vi "EnFlo_Seeder_Control.vi"(0 "Current Time (s)":dbl) -> ()   [LabVIEW 2016]
panel:
  in  "Minium Seeder power setting (Pmin)":dbl=27.0
  in  "Minimum Transducer Setting (Tmin)":dbl=6.0
  in  "Fluid Flowrate Factor":dbl=1.2 min=0.2 max=4.0 step=0.1 format="%.1g"
  in  "Sugar Strength":dbl=0.23
  out "Leak Detected or Emergency Stop":bool
  in  "Performing hand clean":bool
  out "Run Transducer":bool
  out "Sugar Pump":bool
  out "Low Flow":bool
  out "High Flow":bool
  out "Time Since Last Flush (min)":dbl
  out "Running Flush time":dbl
  out "Transducer setting":dbl
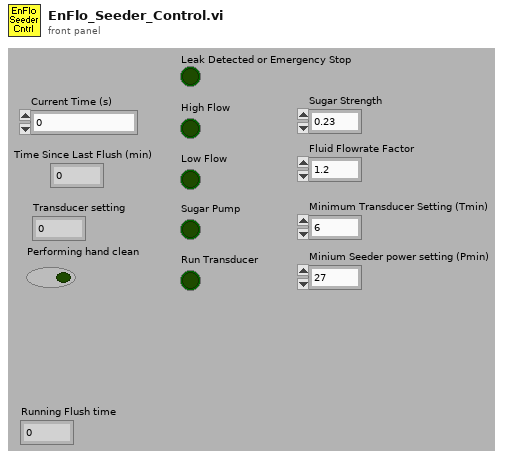
[diagram p1: front panel]
types:
  T1 = typedef "LVDateTimeRec.ctl" = cluster{"fractional second":dbl, "second":i32, "minute":i32, "hour":i32, "day of month":i32, "month":i32, "year":i32, "day of week":i32, "day of year":i32, "DST":i32}
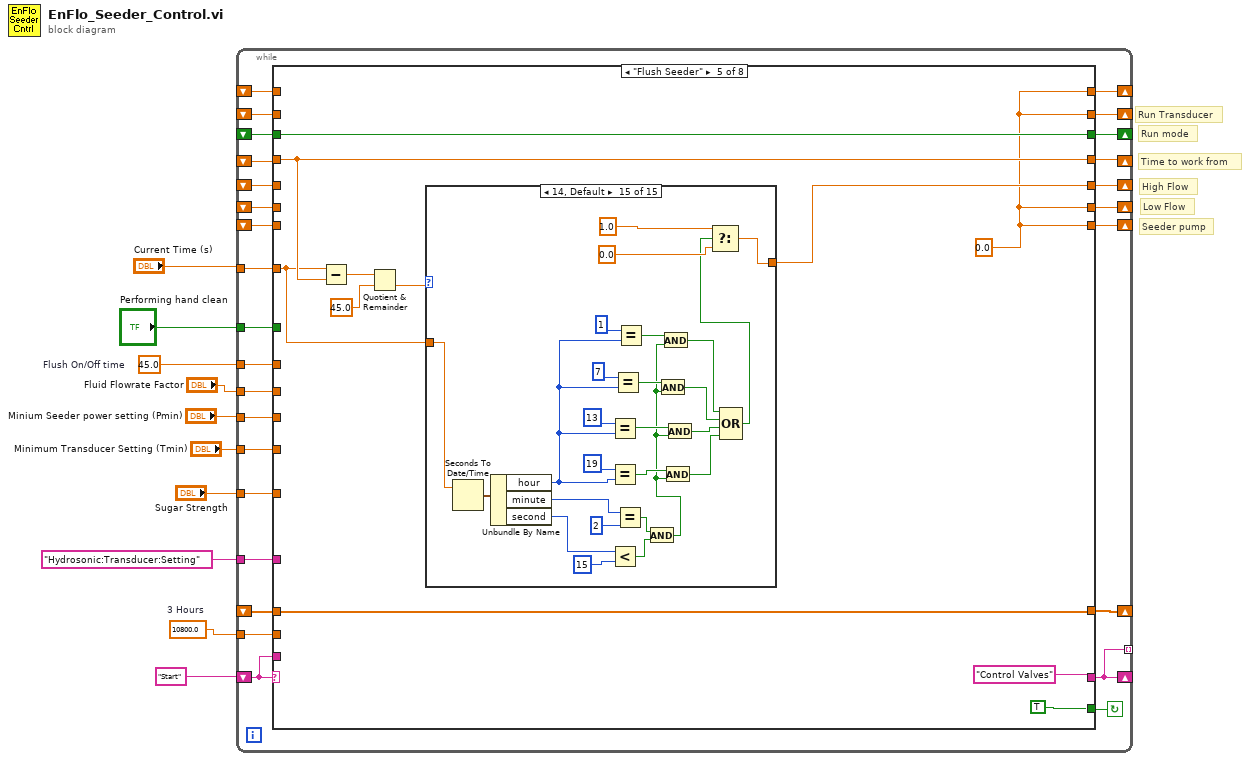
[diagram p0: block diagram]
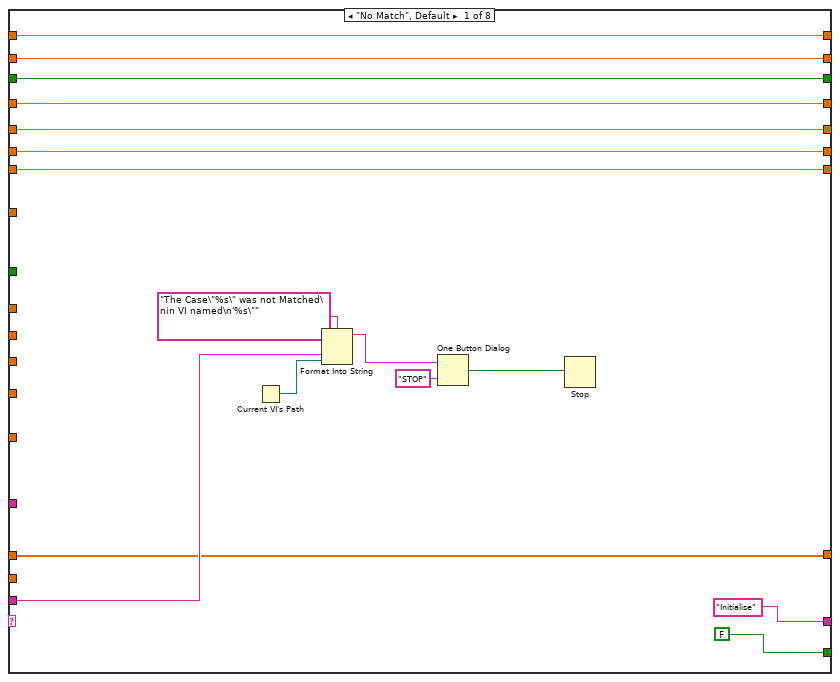
[diagram p2: hidden frame]
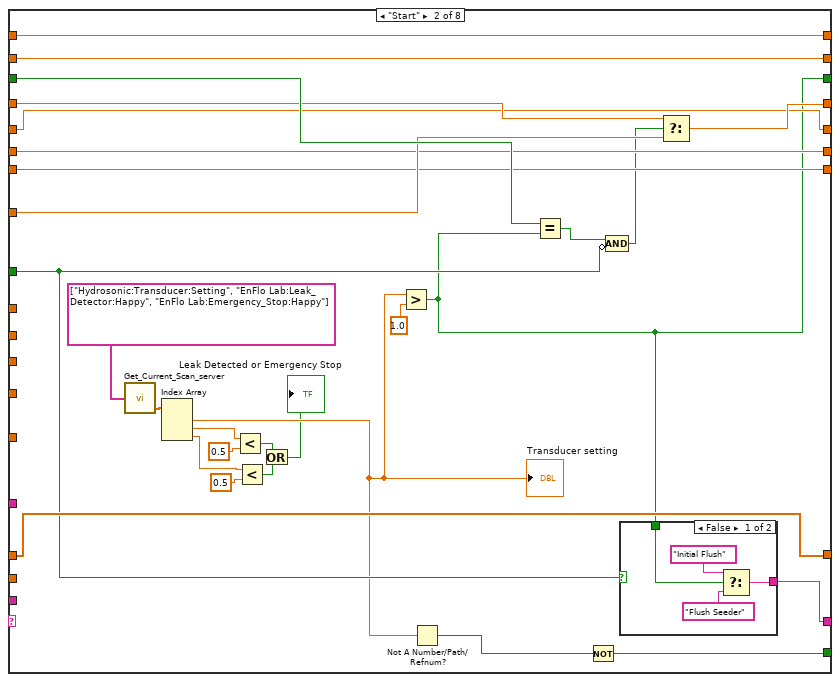
[diagram p3: hidden frame]
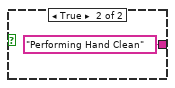
[diagram p4: hidden frame]
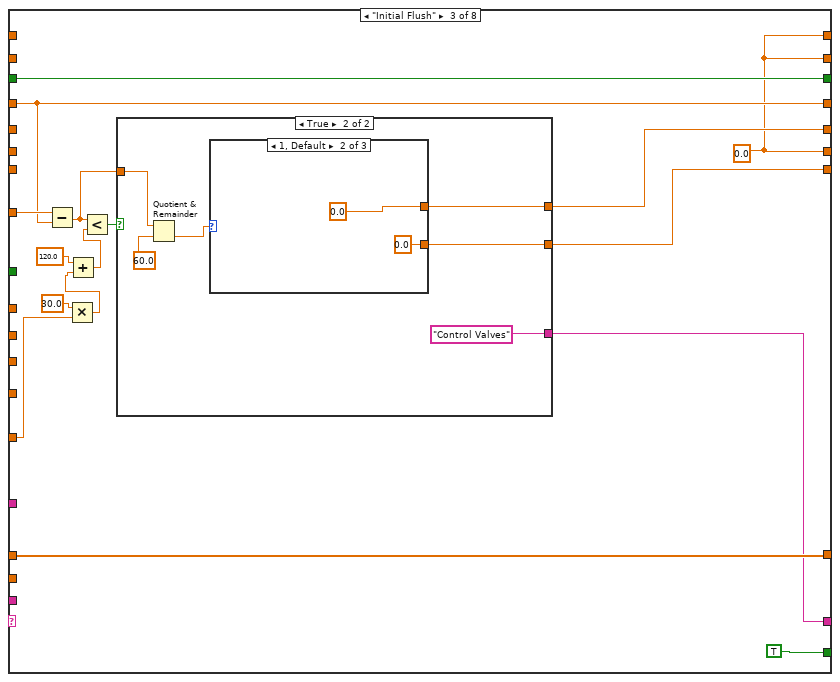
[diagram p5: hidden frame]
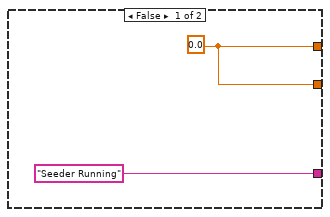
[diagram p6: hidden frame]
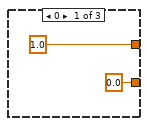
[diagram p7: hidden frame]
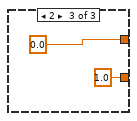
[diagram p8: hidden frame]
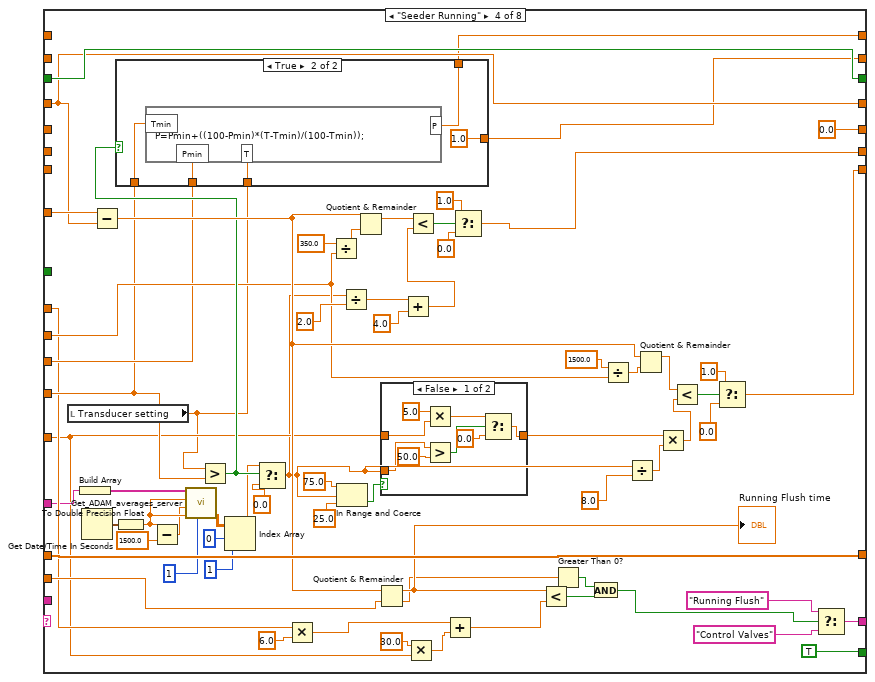
[diagram p9: hidden frame]
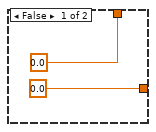
[diagram p11: hidden frame]
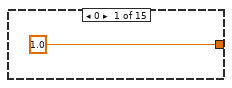
[diagram p12: hidden frame]
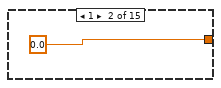
[diagram p13: hidden frame]
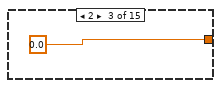
[diagram p14: hidden frame]
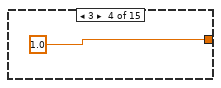
[diagram p15: hidden frame]
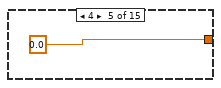
[diagram p16: hidden frame]
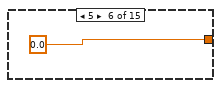
[diagram p17: hidden frame]
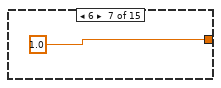
[diagram p18: hidden frame]
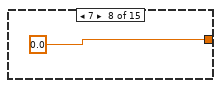
[diagram p19: hidden frame]
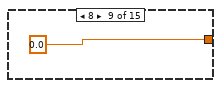
[diagram p20: hidden frame]
diagram:
  w2 = 45.0  # Flush On/Off time
  w8 = 10800.0  # 3 Hours
  # "Run Transducer"
  # "Seeder pump"
  # "Low Flow"
  # "High Flow"
  # "Run mode"
  # "Time to work from"
  n1 = while {
    shift-left: "Start" -> [w37]
    shift-right: [w21] -> _
    shift-right: [w36] -> _
    shift-left: _ -> [w33]
    shift-right: [w35] -> _
    shift-left: _ -> [w34]
    tunnel: "Current Time (s)" -> [w32]
    shift-right: [w30] -> _
    shift-left: _ -> [w31]
    shift-right: [w29] -> _
    shift-left: _ -> [w28]
    shift-right: [w26] -> _
    shift-left: _ -> [w27]
    shift-right: [w24] -> _
    shift-left: _ -> [w25]
    shift-right: [w23] -> _
    shift-left: _ -> [w22]
    tunnel: [w21] -> _ mode=indexing
    tunnel: w8 -> [w20]
    tunnel: "Performing hand clean" -> [w19]
    tunnel: "Sugar Strength" -> [w18]
    shift-right: [w17] -> _
    shift-left: _ -> [w16]
    tunnel: "Fluid Flowrate Factor" -> [w15]
    tunnel: "Minimum Transducer Setting (Tmin)" -> [w14]
    tunnel: "Minium Seeder power setting (Pmin)" -> [w13]
    tunnel: w2 -> [w12]
    tunnel: "Hydrosonic:Transducer:Setting" -> [w11]
    stop <- w38 continue-if-true
    n2 = case shown="\"Flush Seeder\"" w37 {
      tunnel: [FALSE w80 TRUE TRUE TRUE TRUE TRUE FALSE] -> w38
      tunnel: ["Initialise" w75 w94 w164 "Control Valves" "Control Valves" "Control Valves" "End"] -> w21
      tunnel: w37 -> [w49 _ _ _ _ _ _ _]
      tunnel: [w44 w78 w97 w183 w209 w255 w269 w322] -> w36
      tunnel: [w46 w60 w102 w185 w210 w256 w270 w331] -> w35
      tunnel: w34 -> [w46 w79 w102 w185 w210 w256 w270 w331]
      tunnel: w33 -> [w44 w77 w97 w183 w209 w255 w269 w322]
      tunnel: w32 -> [_ w76 w98 w184 w202 _ _ w323]
      tunnel: w31 -> [w45 w74 _ _ _ _ _ w319]
      tunnel: [w45 w74 w101 0.0 w205 w253 w268 w319] -> w30
      tunnel: w28 -> [w43 w72 _ _ _ _ _ w317]
      tunnel: [w43 w72 w88 w173 w203 w253 w264 w317] -> w29
      tunnel: w27 -> [w42 w71 _ _ _ _ _ w315]
      tunnel: [w42 w71 w99 w167 w203 w253 w265 w315] -> w26
      tunnel: w25 -> [w41 w73 w100 w182 w204 w254 w267 w311]
      tunnel: [w41 w73 w100 w182 w204 w254 w267 w304] -> w24
      tunnel: w22 -> [w40 w70 _ _ _ _ _ w313]
      tunnel: [w40 w70 w88 w148 w203 w253 w264 w313] -> w23
      tunnel: w20 -> [_ _ _ w156 _ _ _ w307]
      tunnel: w19 -> [_ w67 _ _ _ _ _ _]
      tunnel: w18 -> [_ _ w91 w123 _ _ _ _]
      tunnel: [w39 w63 w88 w147 w203 w253 w264 w299] -> w17
      tunnel: w16 -> [w39 w63 _ _ _ _ _ w299]
      tunnel: w15 -> [_ _ _ w142 _ _ _ _]
      tunnel: w14 -> [_ _ _ w139 _ _ _ _]
      tunnel: w13 -> [_ _ _ w140 _ _ _ _]
      tunnel: w12 -> [_ _ _ w138 _ _ w263 _]
      tunnel: w11 -> [_ _ _ w135 _ _ _ _]
      frame "No Match", Default {
        n3 = Current VI's Path() -> (path=w48:path)
        n4 = Format Into String(format string="The Case\"%s\" was not Matched\nin VI named\n'%s\"" ("Format String"), w49, w48) -> (resulting string=w52:string)  [unwired: 2 in, 1 out]
        n5 = One Button Dialog(message=w52, button name ("OK")="STOP") -> (true=w50:bool)
        n6 = Stop(stop? (T)=w50) -> ()
      }
      frame "Start" {
        n7 = call "Get_Current_Scan_server.vi"("Desired Channels"=string[] ["Hydrosonic:Transducer:Setting", "EnFlo Lab:Leak_Detector:Happy", "EnFlo Lab:Emergency_Stop:Happy"] ("appended array")) -> ("Numerical Values"=w82:dbl[])  [unwired: 2 out]
        n8 = Index Array(array=w82) -> (element #1=w62:dbl, element #2=w65:dbl, element #3=w58:dbl)  [unwired: 3 in]
        "Transducer setting" <- w62
        n9 = Less?(x=w65, y=0.5) -> (x < y?=w56:bool)
        n10 = Less?(x=w58, y=0.5) -> (x < y?=w57:bool)
        n11 = Or(x=w56, y=w57) -> (x .or. y?=→"Leak Detected or Emergency Stop":bool)
        n12 = Greater?(x=w62, y=1.0) -> (0:w60:bool)
        n13 = Not A Number/Path/Refnum?(number/path/refnum=w62) -> (NaN/Path/Refnum?=w81:bool)
        n14 = Equal?(x=w79, y=w60) -> (x = y?=w69:bool)
        n15 = Not(x=w81) -> (.not. x?=w80:bool)
        n16 = Compound Arithmetic op=AND(w69, invert w67) -> (w68:bool)
        n17 = case shown="False" w67 {
          tunnel: w60 -> [w86 _]
          tunnel: [w85 "Performing Hand Clean"] -> w75
          frame False {
            n18 = Select(t="Initial Flush", s=w86, f="Flush Seeder") -> (s? t:f=w85:string)
          }
          frame True {
          }
        }
        n19 = Select(t=w77, s=w68, f=w76) -> (s? t:f=w78:dbl)
      }
      frame "Initial Flush" {
        w88 = 0.0
        n20 = Subtract(x=w98, y=w97) -> (x-y=w95:dbl)
        n21 = Multiply(x=30.0 ("y"), y=w91) -> (x*y=w90:dbl)
        n22 = Add(x=120.0 ("y"), y=w90) -> (x+y=w89:dbl)
        n23 = Less?(x=w95, y=w89) -> (x < y?=w96:bool)
        n24 = case shown="True" w96 {
          tunnel: [w105 w111] -> w101
          tunnel: [w105 w110] -> w99
          tunnel: w95 -> [_ w108]
          tunnel: ["Seeder Running" "Control Valves"] -> w94
          frame False {
            w105 = 0.0
          }
          frame True {
            n25 = Quotient & Remainder(x=w108, y=60.0) -> (floor(x/y)=w107:dbl)  [unwired: 1 out]
            n26 = case shown="1, Default" w107 {
              tunnel: [1.0 0.0 0.0] -> w111
              tunnel: [0.0 0.0 1.0] -> w110
              frame 0 {
              }
              frame 1, Default {
              }
              frame 2 {
              }
            }
          }
        }
      }
      frame "Seeder Running" {
        n27 = local read "Transducer setting"() -> (w118:dbl)
        n28 = Build Array(w135) -> (w134:string[])
        n29 = Get Date/Time In Seconds() -> (seconds since 1Jan1904=w133:timestamp)
        n30 = Subtract(x=w184, y=w183) -> (x-y=w162:dbl)
        n31 = To Double Precision Float(number=w133) -> (double precision float=w132:dbl)
        n32 = Subtract(x=w132, y=1500.0) -> (x-y=w119:dbl)
        n33 = call "Get_ADAM_averages_server.vi"("No of averages"=1, "End time"=w132, "Start time"=w119, "Clients time"=w132, "ADAM Ch Names"=w134) -> ("DBL values"=w130:dbl[][])  [unwired: 1 in, 4 out]
        n34 = Greater?(x=w118, y=w139) -> (0:w149:bool)
        n35 = case shown="True" w149 {
          tunnel: [0.0 1.0] -> w148
          tunnel: [0.0 w198] -> w147
          tunnel: w140 -> [_ w200]
          tunnel: w139 -> [_ w199]
          tunnel: w118 -> [_ w197]
          frame False {
          }
          frame True {
            n36 = formula code="P=Pmin+((100-Pmin)*(T-Tmin)/(100-Tmin));"("Tmin"=w199, "T"=w197, "Pmin"=w200) -> ("P"=w198:dbl)
          }
        }
        n37 = Index Array(array=w130, index (row)=0, index (col)=1 ("disabled index (col)")) -> (element=w127:dbl)
        n38 = Select(t=w127, s=w149, f=0.0) -> (s? t:f=w121:dbl)
        n39 = Multiply(x=w138, y=6.0) -> (x*y=w136:dbl)
        n40 = Divide(x=350.0 ("y"), y=w142) -> (x/y=w144:dbl)
        n41 = In Range and Coerce(upper limit=75.0, x=w121, lower limit=25.0) -> (In Range?=w124:bool)  [unwired: 1 out]
        n42 = Divide(x=w121, y=2.0) -> (x/y=w146:dbl)
        n43 = Quotient & Remainder(x=w162, y=w144) -> (x-y*floor(x/y)=w181:dbl)  [unwired: 1 out]
        n44 = Quotient & Remainder(x=w162, y=w156) -> (x-y*floor(x/y)=w163:dbl, floor(x/y)=w160:dbl)
        "Running Flush time" <- w163
        n45 = case shown="False" w124 {
          tunnel: w123 -> [w187 w194]
          tunnel: [w191 w194] -> w122
          tunnel: w121 -> [w193 _]
          frame False {
            n46 = Multiply(x=5.0, y=w187) -> (x*y=w188:dbl)
            n47 = Greater?(x=w193, y=50.0) -> (0:w190:bool)
            n48 = Select(t=w188, s=w190, f=0.0) -> (s? t:f=w191:dbl)
          }
          frame True {
          }
        }
        n49 = Add(x=w146, y=4.0) -> (x+y=w176:dbl)
        n50 = Multiply(x=30.0 ("y"), y=w123) -> (x*y=w152:dbl)
        n51 = Less?(x=w181, y=w176) -> (x < y?=w180:bool)
        n52 = Add(x=w136, y=w152) -> (x+y=w151:dbl)
        n53 = Select(t=1.0, s=w180, f=0.0) -> (s? t:f=w173:dbl)
        n54 = Less?(x=w163, y=w151) -> (x < y?=w158:bool)
        n55 = Greater Than 0?(x=w160) -> (x > 0?=w159:bool)
        n56 = And(x=w159, y=w158) -> (x .and. y?=w157:bool)
        n57 = Divide(x=1500.0 ("y"), y=w142) -> (x/y=w141:dbl)
        n58 = Divide(x=w121, y=8.0) -> (x/y=w154:dbl)
        n59 = Quotient & Remainder(x=w162, y=w141) -> (x-y*floor(x/y)=w168:dbl)  [unwired: 1 out]
        n60 = Multiply(x=w122, y=w154) -> (x*y=w155:dbl)
        n61 = Less?(x=w168, y=w155) -> (x < y?=w169:bool)
        n62 = Select(t=1.0, s=w169, f=0.0) -> (s? t:f=w167:dbl)
        n63 = Select(t="Running Flush", s=w157, f="Control Valves") -> (s? t:f=w164:string)
      }
      frame "Flush Seeder" {
        w203 = 0.0
        n64 = Subtract(x=w202, y=w209) -> (x-y=w208:dbl)
        n65 = Quotient & Remainder(x=w208, y=45.0) -> (floor(x/y)=w206:dbl)  [unwired: 1 out]
        n66 = case shown="14, Default" w206 {
          tunnel: [1.0 0.0 0.0 1.0 0.0 0.0 1.0 0.0 0.0 1.0 0.0 0.0 1.0 0.0 w249] -> w205
          tunnel: w202 -> [_ _ _ _ _ _ _ _ _ _ _ _ _ _ w252]
          frame 0 {
          }
          frame 1 {
          }
          frame 2 {
          }
          frame 3 {
          }
          frame 4 {
          }
          frame 5 {
          }
          frame 6 {
          }
          frame 7 {
          }
          frame 8 {
          }
          frame 9 {
          }
          frame 10 {
          }
          frame 11 {
          }
          frame 12 {
          }
          frame 13 {
          }
          frame 14, Default {
            n67 = Seconds To Date/Time(time stamp (now)=w252) -> (date time rec=w248:T1)  [unwired: 1 in]
            n68 = Unbundle By Name(w248) -> ("hour"=w229:i32, "minute"=w246:i32, "second"=w244:i32)
            n69 = Equal?(x=13, y=w229) -> (x = y?=w236:bool)
            n70 = Equal?(x=19, y=w229) -> (x = y?=w238:bool)
            n71 = Less?(x=w244, y=15) -> (x < y?=w241:bool)
            n72 = Equal?(x=7, y=w229) -> (x = y?=w237:bool)
            n73 = Equal?(x=w246, y=2) -> (x = y?=w242:bool)
            n74 = Equal?(x=1, y=w229) -> (x = y?=w231:bool)
            n75 = And(x=w242, y=w241) -> (x .and. y?=w228:bool)
            n76 = And(x=w237, y=w228) -> (x .and. y?=w233:bool)
            n77 = And(x=w231, y=w228) -> (x .and. y?=w227:bool)
            n78 = And(x=w238, y=w228) -> (x .and. y?=w235:bool)
            n79 = And(x=w236, y=w228) -> (x .and. y?=w234:bool)
            n80 = Compound Arithmetic op=OR(w227, w233, w234, w235) -> (w232:bool)
            n81 = Select(t=1.0, s=w232, f=0.0) -> (s? t:f=w249:dbl)
          }
        }
      }
      frame "Performing Hand Clean" {
        w253 = 0.0
      }
      frame "Running Flush" {
        w264 = 0.0
        n82 = local read "Running Flush time"() -> (w266:dbl)
        n83 = Quotient & Remainder(x=w266, y=w263) -> (floor(x/y)=w262:dbl)  [unwired: 1 out]
        n84 = To Long Integer(number=w262) -> (32bit integer=w259:i32)
        n85 = feedback-in #1(w259) -> ()
        n86 = feedback #1() -> (w261:i32)  [unwired: 1 in]
        n87 = Not Equal?(x=w259, y=w261) -> (x != y?=w260:bool)
        n88 = case shown="2" w259 {
          tunnel: [1.0 0.0 1.0 0.0 1.0 0.0 0.0] -> w268
          tunnel: [0.0 0.0 0.0 0.0 0.0 0.0 1.0] -> w265
          tunnel: w260 -> [_ _ _ _ _ _ w285]
          frame 0 {
          }
          frame 1 {
          }
          frame 2 {
          }
          frame 3 {
          }
          frame 4 {
          }
          frame 5, Default {
          }
          frame 6 {
            n89 = local read "Transducer setting"() -> (w288:dbl)
            n90 = In Range and Coerce(upper limit=90.0, x=w288, lower limit=8.0) -> (In Range?=w286:bool)  [unwired: 1 out]
            n91 = And(x=w286, y=w285) -> (x .and. y?=w287:bool)
            n92 = case shown="True" w287 {
              tunnel: w288 -> [_ w296]
              frame False {
              }
              frame True {
                n93 = Add(x=w296, y=10.0) -> (x+y=w293:dbl)
                n94 = Build Array("Hydrosonic:Transducer:Setting") -> (w297:string[])
                n95 = Build Array(w293) -> (w294:dbl[])
                n96 = call "ASYNC_Adam_server.vi"("Values"=w294, "Channel Names"=w297) -> ()  [unwired: 1 in, 3 out]
              }
            }
          }
        }
      }
      frame "Control Valves" {
        n97 = Subtract(x=w323, y=w322) -> (x-y=w308:dbl)
        n98 = local read "Leak Detected or Emergency Stop"() -> (w305:bool)
        n99 = Quotient & Remainder(x=w308, y=w307) -> (x-y*floor(x/y)=w306:dbl)  [unwired: 1 out]
        n100 = Divide(x=w306, y=60.0) -> (x/y=→"Time Since Last Flush (min)":dbl)
        n101 = Build Array(w313, w319, w317, w315, w299) -> (w301:dbl[])
        n102 = Array Size(array=w311) -> (size(s)=w310:i32)
        n103 = Equal To 0?(x=w310) -> (x = 0?=w309:bool)
        n104 = Array Size(array=w301) -> (size(s)=w303:i32)
        n105 = Initialize Array(0.0 ("element"), w303) -> (w300:dbl[])
        n106 = Select(t=w300, s=w305, f=w301) -> (s? t:f=w304:dbl[])
        n107 = case shown="False" w309 {
          tunnel: w304 -> [w336 w341]
          tunnel: string[] ["Hydrosonic:Seeder:Enable", "EnFlo_Tunnel:Seeder:High_Flow", "EnFlo_Tunnel:Seeder:Low_Flow", "EnFlo_Tunnel:Seeder_Pump:Enable", "EnFlo_Tunnel:Seeder:Power"] ("Desired Ch Names") -> [w335 w342]
          tunnel: [w334 w342] -> w327
          tunnel: [w333 w341] -> w326
          tunnel: w311 -> [w332 _]
          frame False {
            n108 = for {
              tunnel: w332 -> [w340] mode=indexing
              tunnel: w336 -> [w339] mode=indexing
              tunnel: [w339] -> w333 mode=indexing if=w337
              tunnel: w335 -> [w338] mode=indexing
              tunnel: [w338] -> w334 mode=indexing if=w337
              n109 = Not Equal?(x=w339, y=w340) -> (x != y?=w337:bool)
            }
          }
          frame True {
          }
        }
        n110 = Array Size(array=w326) -> (size(s)=w330:i32)
        n111 = Greater Than 0?(x=w330) -> (x > 0?=w329:bool)
        n112 = case shown="True" w329 {
          tunnel: w326 -> [_ w344]
          tunnel: w327 -> [_ w343]
          frame False {
          }
          frame True {
            n113 = call "ASYNC_Adam_server.vi"("Values"=w344, "Channel Names"=w343) -> ()  [unwired: 1 in, 3 out]
          }
        }
        n114 = Greater Than 0?(x=w319) -> (x > 0?=→"High Flow":bool)
        n115 = Greater Than 0?(x=w317) -> (x > 0?=→"Low Flow":bool)
        n116 = Greater Than 0?(x=w313) -> (x > 0?=→"Run Transducer":bool)
        n117 = Greater Than 0?(x=w315) -> (x > 0?=→"Sugar Pump":bool)
      }
    }
  }
